vi "Durchflussanpassung neuer Sensor.vi"(8 "Offset":sgl, 9 "Endpunkt":sgl, 11 "Eingang":sgl) -> (3 "Ausgang":dbl)   [LabVIEW 2020, in "Allgemein.lvlib"]
uses:
  Allgemein.lvlib
panel:
  # "mit Seitenausgang"
  # "Bohrung 3.7mm"
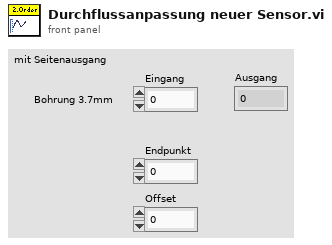
[diagram p1: front panel]
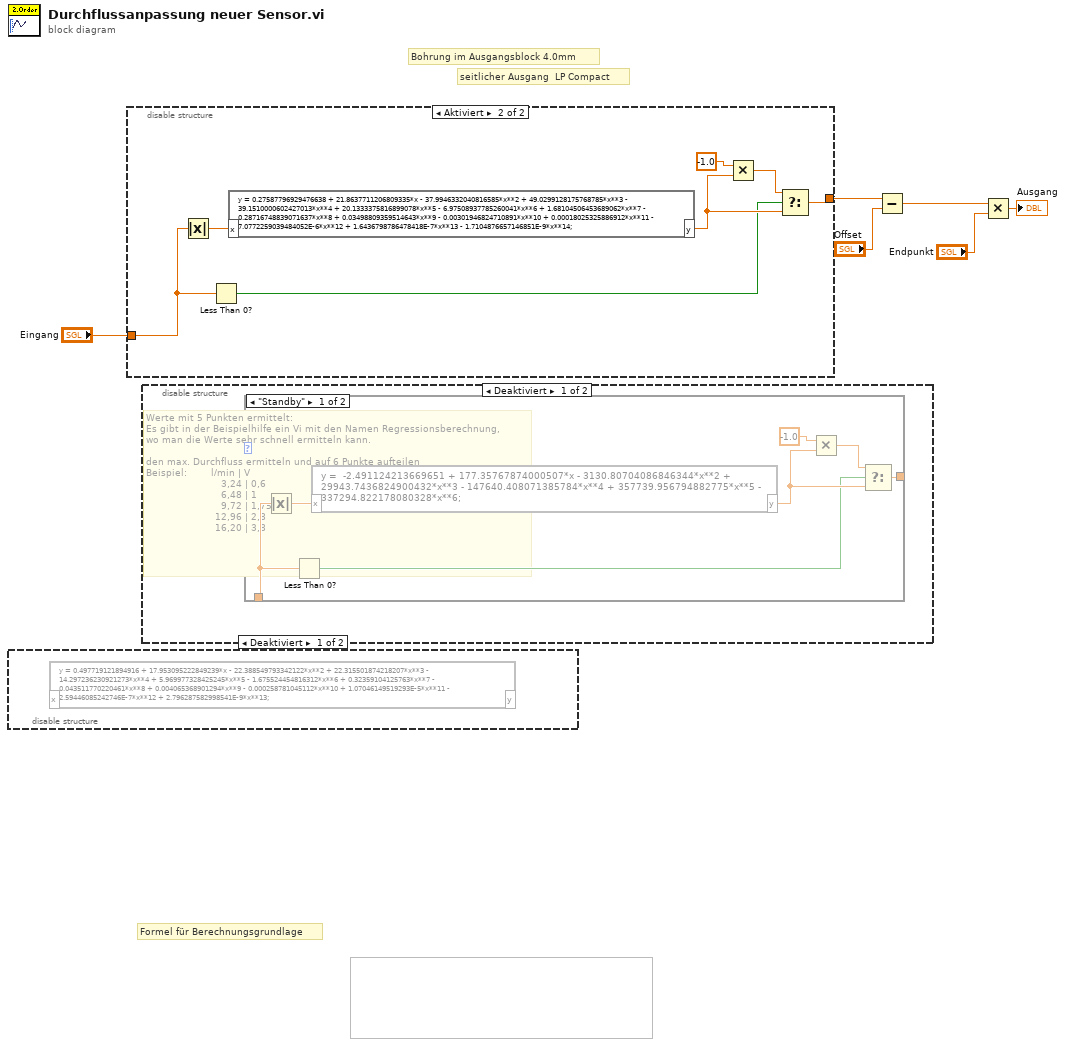
[diagram p0: block diagram]
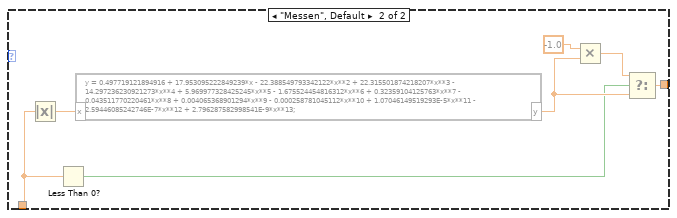
[diagram p3: hidden frame]
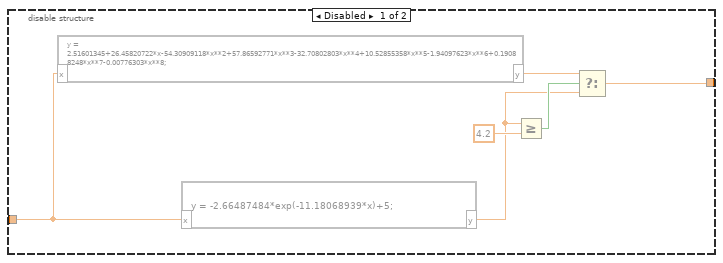
[diagram p5: hidden frame]
diagram:
  # "seitlicher Ausgang  LP Compact"
  # "Bohrung im Ausgangsblock 4.0mm"
  # "Formel für Berechnungsgrundlage"
  n1 = disable-structure shown="Deaktiviert" {
    frame Disabled {
      n2 = formula code="y = 0.497719121894916 + 17.953095222849239*x - 22.388549793342122*x**2 + 22.315501874218207*x**3 - 14.297236230921273*x**4 + 5.969977328425245*x**5 - 1.675524454816312*x**6 + 0.32359104125763*x**7 - 0.043511770220461*x**8 + 0.004065368901294*x**9 - 0.000258781045112*x**10 + 1.07046149519293E-5*x**11 - 2.59446085242746E-7*x**12 + 2.796287582998541E-9*x**13;"() -> ()  [unwired: 1 in, 1 out]
    }
    frame Enabled {
    }
  }
  n3 = disable-structure shown="Aktiviert" {
    disable-tunnel: "Eingang" -> [w12 w19]
    disable-tunnel: [w9 w18] -> w1
    frame Disabled {
      n4 = formula code="y = 2.51601345+26.45820722*x-54.30909118*x**2+57.86592771*x**3-32.70802803*x**4+10.52855358*x**5-1.94097623*x**6+0.19088248*x**7-0.00776303*x**8;"("x"=w12) -> ("y"=w8:dbl)
      n5 = formula code="y = -2.66487484*exp(-11.18068939*x)+5;"("x"=w12) -> ("y"=w7:dbl)
      n6 = Greater Or Equal?(x=w7, y=4.2) -> (x >= y?=w10:bool)
      n7 = Select(t=w8, s=w10, f=w7) -> (s? t:f=w9:dbl)
    }
    frame Enabled {
      n8 = Absolute Value(x=w19) -> (abs(x)=w17:sgl)
      n9 = Less Than 0?(x=w19) -> (x < 0?=w13:bool)
      n10 = formula code="y = 0.27587796929476638 + 21.8637711206809335*x - 37.9946332040816585*x**2 + 49.0299128175768785*x**3 - 39.1510000602427013*x**4 + 20.1333375816899078*x**5 - 6.97508937785260041*x**6 + 1.68104506453689062*x**7 - 0.28716748839071637*x**8 + 0.03498809359514643*x**9 - 0.00301946824710891*x**10 + 0.00018025325886912*x**11 - 7.0772259039484052E-6*x**12 + 1.6436798786478418E-7*x**13 - 1.7104876657146851E-9*x**14;"("x"=w17) -> ("y"=w14:dbl)
      n11 = Multiply(x=-1.0 ("y"), y=w14) -> (x*y=w15:dbl)
      n12 = Select(t=w15, s=w13, f=w14) -> (s? t:f=w18:dbl)
    }
  }
  n13 = disable-structure shown="Deaktiviert" {
    frame Disabled {
      # "Werte mit 5 Punkten ermittelt:\nEs gibt in der Beispielhilfe ein Vi mit den Namen Regressionsberechnung,\nwo man die Werte sehr schnell ermitteln kann.\n\nden max. Durchfluss ermitteln und auf 6 Punkte aufteilen\nBeispiel:        l/min | V\n                         3,24 | 0,6\n                         6,48 | 1\n                         9,72 | 1,75\n                       12,96 | 2,8\n                       16,20 | 3,8"
      n14 = case shown="\"Standby\"" {
        selector: _ -> [_ _]
        tunnel: _ -> [w25 w32]
        tunnel: [w23 w30] -> _
        frame "Standby" {
          n15 = Absolute Value(x=w25) -> (abs(x)=w26:dbl)
          n16 = Less Than 0?(x=w25) -> (x < 0?=w20:bool)
          n17 = formula code="y =  -2.491124213669651 + 177.35767874000507*x - 3130.80704086846344*x**2 + 29943.7436824900432*x**3 - 147640.408071385784*x**4 + 357739.956794882775*x**5 - 337294.822178080328*x**6;"("x"=w26) -> ("y"=w21:dbl)
          n18 = Multiply(x=-1.0 ("y"), y=w21) -> (x*y=w22:dbl)
          n19 = Select(t=w22, s=w20, f=w21) -> (s? t:f=w23:dbl)
        }
        frame "Messen", Default {
          n20 = Absolute Value(x=w32) -> (abs(x)=w33:dbl)
          n21 = Less Than 0?(x=w32) -> (x < 0?=w27:bool)
          n22 = formula code="y = 0.497719121894916 + 17.953095222849239*x - 22.388549793342122*x**2 + 22.315501874218207*x**3 - 14.297236230921273*x**4 + 5.969977328425245*x**5 - 1.675524454816312*x**6 + 0.32359104125763*x**7 - 0.043511770220461*x**8 + 0.004065368901294*x**9 - 0.000258781045112*x**10 + 1.07046149519293E-5*x**11 - 2.59446085242746E-7*x**12 + 2.796287582998541E-9*x**13;"("x"=w33) -> ("y"=w28:dbl)
          n23 = Multiply(x=-1.0 ("y"), y=w28) -> (x*y=w29:dbl)
          n24 = Select(t=w29, s=w27, f=w28) -> (s? t:f=w30:dbl)
        }
      }
    }
    frame Enabled {
    }
  }
  n25 = Subtract(x=w1, y="Offset") -> (x-y=w4:dbl)
  n26 = Multiply(x=w4, y="Endpunkt") -> (x*y=→"Ausgang":dbl)
